vi "Begin.vi"(8 "error in":errorcluster) -> (0 "error out":errorcluster)   [LabVIEW 2016]
doc: "Called before other user functions, this VI is expected to open initial I/O refnums, load in file data, and do all program initialization. Notice that the <B>error out</B> terminal is simply used for data flow. Wiring it to other structures or subVIs ensures that this VI runs first."
uses:
  <vilib>/Rock Robotics/WPI/DriverStation/WPI_DriverStationRobotMode2.ctl
  <vilib>/Rock Robotics/WPI/Joystick/WPI_JoystickDeviceEnum.ctl
  <vilib>/Rock Robotics/WPI/ThirdParty/CanMotor/TalonSRX/WPI_CANTalonSRX_APIControlMode.ctl
  <vilib>/Rock Robotics/WPI/ThirdParty/CanMotor/TalonSRX/WPI_CANTalonSRX_BrakeOverride.ctl
  <vilib>/Rock Robotics/WPI/ThirdParty/CanMotor/TalonSRX/WPI_CANTalonSRX_APIFeedbackSelect.ctl
  <vilib>/Rock Robotics/WPI/Solenoid/WPI_SolenoidChannel.ctl
  <vilib>/Rock Robotics/WPI/Solenoid/WPI_SolenoidValue.ctl
  <vilib>/Rock Robotics/SystemInterfaces/DIO/FPGA_DIOChannel.ctl
  Robot Global Data.vi
  <vilib>/Rock Robotics/WPI/Solenoid/WPI_SolenoidOpenSingle.vi
  <vilib>/Rock Robotics/WPI/Solenoid/WPI_SolenoidSetEnum.vi
  <vilib>/Rock Robotics/WPI/Switch/WPI_SwitchOpenLimit.vi
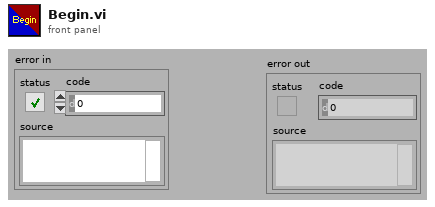
[diagram p1: front panel]
types:
  T1 = typedef "FPGA_DIOChannel.ctl" = enum8{"DIO 0", "DIO 1", "DIO 2", "DIO 3", "DIO 4", "DIO 5", "DIO 6", "DIO 7", "DIO 8", "DIO 9", "DIO MXP 0", "DIO MXP 1", "DIO MXP 2", "DIO MXP 3", "DIO MXP 4", "DIO MXP 5", "DIO MXP 6", "DIO MXP 7", "DIO MXP 8", "DIO MXP 9", "DIO MXP 10", "DIO MXP 11", "DIO MXP 12", "DIO MXP 13", "DIO MXP 14", "DIO MXP 15", "SPI Port CS1", "SPI Port CS2", "SPI Port CS3", "SPI Port MISO", "SPI Port MOSI", "Invalid"}
  T2 = typedef "WPI_SolenoidValue.ctl" = enum16{"Off", "On", "Forward", "Reverse"}
  T3 = typedef "WPI_SolenoidChannel.ctl" = enum8{"Solenoid 0", "Solenoid 1", "Solenoid 2", "Solenoid 3", "Solenoid 4", "Solenoid 5", "Solenoid 6", "Solenoid 7", "Invalid"}
  T4 = typedef "WPI_CANTalonSRX_BrakeOverride.ctl" = enum8{"No Override", "Override to Coast", "Override to Brake"}
  T5 = typedef "WPI_CANTalonSRX_APIControlMode.ctl" = enum8{"Percent VBus", "Speed", "Position", "Slave", "Unchanged / Invalid", "Voltage Compensation", "Current", "Motion Profile", "Motion Magic"}
  T6 = typedef "WPI_CANTalonSRX_APIFeedbackSelect.ctl" = enum16{"Digital Quadrature Encoder", "Analog Potentiometer", "Analog Encoder", "Count on Quad-A (Rising-Edge)", "Count on Quad-A (Falling-Edge)", "CTR Magnetic Enc (Absolute)", "CTR Magnetic Enc (Relative)", "Pulse Width"}
  T7 = typedef "WPI_JoystickDeviceEnum.ctl" = enum16{"USB 0", "USB 1", "USB 2", "USB 3", "USB 4", "USB 5"}
  T8 = typedef "WPI_DriverStationRobotMode2.ctl" = enum16{"Autonomous Disabled", "Autonomous Enabled", "Teleop Disabled", "Teleop Enabled", "Disconnected", "Finish", "Test Disabled", "Test Enabled", "Emergency Stopped"}
  T9 = typedef "WPI_JoystickDevRef.ctl" = cluster{"Device":T7}
  T10 = typedef "WPI_MotorControlDeviceRef.ctl" = cluster{"DeviceStatus":errorcluster, "Type":T11, "PWM":cluster{"PWM Channel":T12, "DeadBand":T13}, "CAN":cluster{"Device Number":u8, "SetOutput VI Ref":variant, "GetOutput VI Ref":variant, "Enable VI Ref":variant, "Disable VI Ref":variant, "Data":variant}, "Invert":bool}
  T11 = typedef "WPI_MotorControlType.ctl" = enum16{"PWM", "CAN"}
  T12 = typedef "FPGA_DIOPWMChannel.ctl" = enum8{"PWM 0", "PWM 1", "PWM 2", "PWM 3", "PWM 4", "PWM 5", "PWM 6", "PWM 7", "PWM 8", "PWM 9", "PWM MXP 0", "PWM MXP 1", "PWM MXP 2", "PWM MXP 3", "PWM MXP 4", "PWM MXP 5", "PWM MXP 6", "PWM MXP 7", "PWM MXP 8", "PWM MXP 9", "Invalid"}
  T13 = typedef "WPI_PWMDeadband.ctl" = cluster{"Name":string, "maxPositivePwm":i32, "minPositivePwm":i32, "centerPwm":i32, "maxNegativePwm":i32, "minNegativePwm":i32, "angularRange":u16}
  T14 = typedef "WPI_SwitchDevRef.ctl" = cluster{"DevStatus":errorcluster, "DIO Channel":T1, "CntIndex":T15, "Normally Closed":bool}
  T15 = typedef "FPGA_CounterCtrSystemIndex.ctl" = enum8{"Ctr 0", "Ctr 1", "Ctr 2", "Ctr 3", "Ctr 4", "Ctr 5", "Ctr 6", "Ctr 7", "Invalid"}
  T16 = typedef "WPI_SolenoidDevRef.ctl" = cluster{"DevStatus":errorcluster, "Pneumatics Control Module":u8, "Forward Solenoid Channel":T3, "Reverse Solenoid Channel":T3}
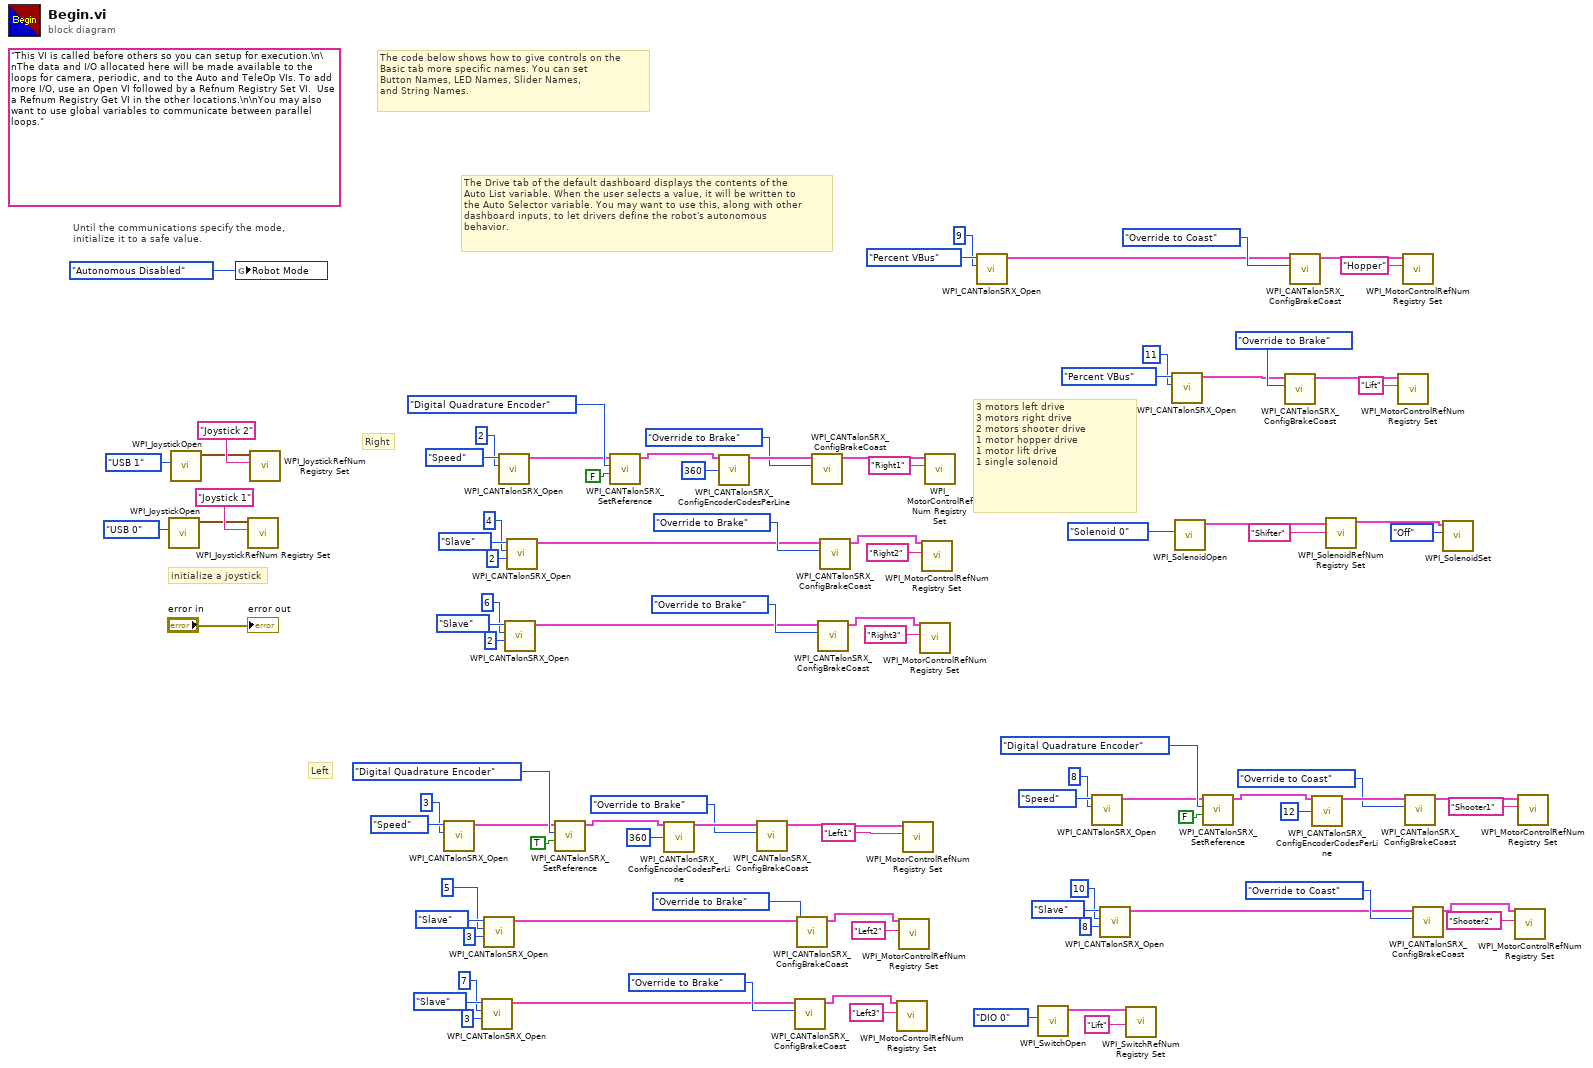
[diagram p0: block diagram]
diagram:
  (unwired) "This VI is called before others so you can setup for execution.\n\nThe data and I/O allocated here will be made available to the loops for camera, periodic, and to the Auto and TeleOp VIs. To add more I/O, use an Open VI followed by a Refnum Registry Set VI.  Use a Refnum Registry Get VI in the other locations.\n\nYou may also want to use global variables to communicate between parallel loops."
  # "3 motors left drive\n3 motors right drive\n2 motors shooter drive\n1 motor hopper drive\n1 motor lift drive\n1 single solenoid"
  # "Right"
  # "Left"
  # "The Drive tab of the default dashboard displays the contents of the\nAuto List variable. When the user selects a value, it will be written to\nthe Auto Selector variable. You may want to use this, along with other\ndashboard inputs, to let drivers define the robot's autonomous\nbehavior."
  # "The code below shows how to give controls on the\nBasic tab more specific names. You can set\nButton Names, LED Names, Slider Names,\nand String Names."
  # "initialize a joystick"
  # "Until the communications specify the mode,\ninitialize it to a safe value."
  n1 = call <vilib>:"WPI_JoystickOpen.vi"("JoystickDevice"=WPI_JoystickDeviceEnum."USB 0") -> ("JoystickDevRef"=w94:T9)  [unwired: 10 in]
  n2 = call <vilib>:"WPI_JoystickOpen.vi"("JoystickDevice"=WPI_JoystickDeviceEnum."USB 1") -> ("JoystickDevRef"=w90:T9)  [unwired: 10 in]
  n3 = global write "Robot Global Data.vi" "Robot Mode"(WPI_DriverStationRobotMode2."Autonomous Disabled" ("Robot Mode")) -> ()
  n4 = call <vilib>:"WPI_JoystickRefNum Registry Set.vi"("refnum name"="Joystick 1", "JoystickDevRef"=w94) -> ()  [unwired: 8 in, 2 out]
  n5 = call <vilib>:"WPI_JoystickRefNum Registry Set.vi"("refnum name"="Joystick 2", "JoystickDevRef"=w90) -> ()  [unwired: 8 in, 2 out]
  n6 = call <vilib>:"WPI_CANTalonSRX_Open.vi"("Device Number"=u8 3, "Control Mode"=WPI_CANTalonSRX_APIControlMode."Speed") -> ("CAN Talon SRX Ref"=w15:T10)  [unwired: 8 in, 1 out]
  n7 = call <vilib>:"WPI_CANTalonSRX_Open.vi"("Master Device Number"=u8 3, "Device Number"=u8 7, "Control Mode"=WPI_CANTalonSRX_APIControlMode."Slave") -> ("CAN Talon SRX Ref"=w66:T10)  [unwired: 7 in, 1 out]
  n8 = call <vilib>:"WPI_CANTalonSRX_Open.vi"("Master Device Number"=u8 3, "Device Number"=u8 5, "Control Mode"=WPI_CANTalonSRX_APIControlMode."Slave") -> ("CAN Talon SRX Ref"=w73:T10)  [unwired: 7 in, 1 out]
  n9 = call <vilib>:"WPI_CANTalonSRX_Open.vi"("Device Number"=u8 2, "Control Mode"=WPI_CANTalonSRX_APIControlMode."Speed") -> ("CAN Talon SRX Ref"=w81:T10)  [unwired: 8 in, 1 out]
  n10 = call <vilib>:"WPI_CANTalonSRX_Open.vi"("Master Device Number"=u8 2, "Device Number"=u8 6, "Control Mode"=WPI_CANTalonSRX_APIControlMode."Slave") -> ("CAN Talon SRX Ref"=w52:T10)  [unwired: 7 in, 1 out]
  n11 = call <vilib>:"WPI_CANTalonSRX_Open.vi"("Master Device Number"=u8 2, "Device Number"=u8 4, "Control Mode"=WPI_CANTalonSRX_APIControlMode."Slave") -> ("CAN Talon SRX Ref"=w59:T10)  [unwired: 7 in, 1 out]
  n12 = call <vilib>:"WPI_CANTalonSRX_SetReference.vi"("Reverse Feedback Sensor"=TRUE, "Feedback Reference"=WPI_CANTalonSRX_APIFeedbackSelect."Digital Quadrature Encoder", "CAN Talon SRX Ref"=w15) -> ("CAN Talon SRX Ref"=w14:T10)  [unwired: 7 in, 1 out]
  n13 = call <vilib>:"WPI_CANTalonSRX_SetReference.vi"("Reverse Feedback Sensor"=FALSE, "Feedback Reference"=WPI_CANTalonSRX_APIFeedbackSelect."Digital Quadrature Encoder", "CAN Talon SRX Ref"=w81) -> ("CAN Talon SRX Ref"=w80:T10)  [unwired: 7 in, 1 out]
  n14 = call <vilib>:"WPI_CANTalonSRX_ConfigEncoderCodesPerLine.vi"("CAN Talon SRX Ref"=w14, "Number Encoder Lines\n(Counts Per Rotation)"=u32 360 ("Number Encoder Lines\n(Counts Per Rotation)")) -> ("CAN Talon SRX Ref"=w18:T10)  [unwired: 12 in, 1 out]
  n15 = call <vilib>:"WPI_CANTalonSRX_ConfigEncoderCodesPerLine.vi"("CAN Talon SRX Ref"=w80, "Number Encoder Lines\n(Counts Per Rotation)"=u32 360 ("Number Encoder Lines\n(Counts Per Rotation)")) -> ("CAN Talon SRX Ref"=w84:T10)  [unwired: 12 in, 1 out]
  n16 = call <vilib>:"WPI_CANTalonSRX_ConfigBrakeCoast.vi"("Brake / Coast Mode"=WPI_CANTalonSRX_BrakeOverride."Override to Brake", "CAN Talon SRX Ref"=w18) -> ("CAN Talon SRX Ref"=w13:T10)  [unwired: 8 in, 1 out]
  n17 = call <vilib>:"WPI_CANTalonSRX_ConfigBrakeCoast.vi"("Brake / Coast Mode"=WPI_CANTalonSRX_BrakeOverride."Override to Brake", "CAN Talon SRX Ref"=w66) -> ("CAN Talon SRX Ref"=w67:T10)  [unwired: 8 in, 1 out]
  n18 = call <vilib>:"WPI_CANTalonSRX_ConfigBrakeCoast.vi"("Brake / Coast Mode"=WPI_CANTalonSRX_BrakeOverride."Override to Brake", "CAN Talon SRX Ref"=w73) -> ("CAN Talon SRX Ref"=w74:T10)  [unwired: 8 in, 1 out]
  n19 = call <vilib>:"WPI_CANTalonSRX_ConfigBrakeCoast.vi"("Brake / Coast Mode"=WPI_CANTalonSRX_BrakeOverride."Override to Brake", "CAN Talon SRX Ref"=w84) -> ("CAN Talon SRX Ref"=w79:T10)  [unwired: 8 in, 1 out]
  n20 = call <vilib>:"WPI_CANTalonSRX_ConfigBrakeCoast.vi"("Brake / Coast Mode"=WPI_CANTalonSRX_BrakeOverride."Override to Brake", "CAN Talon SRX Ref"=w52) -> ("CAN Talon SRX Ref"=w53:T10)  [unwired: 8 in, 1 out]
  n21 = call <vilib>:"WPI_CANTalonSRX_ConfigBrakeCoast.vi"("Brake / Coast Mode"=WPI_CANTalonSRX_BrakeOverride."Override to Brake", "CAN Talon SRX Ref"=w59) -> ("CAN Talon SRX Ref"=w60:T10)  [unwired: 8 in, 1 out]
  n22 = call <vilib>:"WPI_MotorControlRefNum Registry Set.vi"("refnum name"="Left3", "MotorControlDevRef"=w67) -> ()  [unwired: 8 in, 2 out]
  n23 = call <vilib>:"WPI_MotorControlRefNum Registry Set.vi"("refnum name"="Left2", "MotorControlDevRef"=w74) -> ()  [unwired: 8 in, 2 out]
  n24 = call <vilib>:"WPI_MotorControlRefNum Registry Set.vi"("refnum name"="Left1", "MotorControlDevRef"=w13) -> ()  [unwired: 8 in, 2 out]
  n25 = call <vilib>:"WPI_MotorControlRefNum Registry Set.vi"("refnum name"="Right3", "MotorControlDevRef"=w53) -> ()  [unwired: 8 in, 2 out]
  n26 = call <vilib>:"WPI_MotorControlRefNum Registry Set.vi"("refnum name"="Right2", "MotorControlDevRef"=w60) -> ()  [unwired: 8 in, 2 out]
  n27 = call <vilib>:"WPI_MotorControlRefNum Registry Set.vi"("refnum name"="Right1", "MotorControlDevRef"=w79) -> ()  [unwired: 8 in, 2 out]
  n28 = call <vilib>:"WPI_CANTalonSRX_Open.vi"("Device Number"=u8 9, "Control Mode"=WPI_CANTalonSRX_APIControlMode."Percent VBus") -> ("CAN Talon SRX Ref"=w10:T10)  [unwired: 8 in, 1 out]
  n29 = call-poly <vilib>:"WPI_SwitchOpen.vi"("DIO Channel"=FPGA_DIOChannel."DIO 0") -> ("SwitchDevRef"=w2:T14)  [unwired: 9 in, 1 out]
  n30 = call <vilib>:"WPI_CANTalonSRX_Open.vi"("Device Number"=u8 8, "Control Mode"=WPI_CANTalonSRX_APIControlMode."Speed") -> ("CAN Talon SRX Ref"=w43:T10)  [unwired: 8 in, 1 out]
  n31 = call <vilib>:"WPI_CANTalonSRX_Open.vi"("Master Device Number"=u8 8, "Device Number"=u8 10, "Control Mode"=WPI_CANTalonSRX_APIControlMode."Slave") -> ("CAN Talon SRX Ref"=w34:T10)  [unwired: 7 in, 1 out]
  n32 = call <vilib>:"WPI_SwitchRefNum Registry Set.vi"("refnum name"="Lift", "SwitchDevRef"=w2) -> ()  [unwired: 8 in, 2 out]
  n33 = call <vilib>:"WPI_CANTalonSRX_Open.vi"("Device Number"=u8 11, "Control Mode"=WPI_CANTalonSRX_APIControlMode."Percent VBus") -> ("CAN Talon SRX Ref"=w9:T10)  [unwired: 8 in, 1 out]
  n34 = call-poly <vilib>:"WPI_SolenoidOpen.vi"("Solenoid Channel"=WPI_SolenoidChannel."Solenoid 0") -> ("SolenoidDevRef"=w7:T16)  [unwired: 9 in, 1 out]
  n35 = call <vilib>:"WPI_CANTalonSRX_SetReference.vi"("Reverse Feedback Sensor"=FALSE, "Feedback Reference"=WPI_CANTalonSRX_APIFeedbackSelect."Digital Quadrature Encoder", "CAN Talon SRX Ref"=w43) -> ("CAN Talon SRX Ref"=w42:T10)  [unwired: 7 in, 1 out]
  n36 = call <vilib>:"WPI_CANTalonSRX_ConfigBrakeCoast.vi"("Brake / Coast Mode"=WPI_CANTalonSRX_BrakeOverride."Override to Brake", "CAN Talon SRX Ref"=w9) -> ("CAN Talon SRX Ref"=w24:T10)  [unwired: 8 in, 1 out]
  n37 = call <vilib>:"WPI_CANTalonSRX_ConfigBrakeCoast.vi"("Brake / Coast Mode"=WPI_CANTalonSRX_BrakeOverride."Override to Coast", "CAN Talon SRX Ref"=w10) -> ("CAN Talon SRX Ref"=w29:T10)  [unwired: 8 in, 1 out]
  n38 = call <vilib>:"WPI_CANTalonSRX_ConfigEncoderCodesPerLine.vi"("CAN Talon SRX Ref"=w42, "Number Encoder Lines\n(Counts Per Rotation)"=u32 12 ("Number Encoder Lines\n(Counts Per Rotation)")) -> ("CAN Talon SRX Ref"=w46:T10)  [unwired: 12 in, 1 out]
  n39 = call <vilib>:"WPI_SolenoidRefNum Registry Set.vi"("refnum name"="Shifter", "SolenoidDevRef"=w7) -> ("SolenoidDevRef"=w6:T16)  [unwired: 8 in, 1 out]
  n40 = call <vilib>:"WPI_MotorControlRefNum Registry Set.vi"("refnum name"="Lift", "MotorControlDevRef"=w24) -> ()  [unwired: 8 in, 2 out]
  n41 = call <vilib>:"WPI_MotorControlRefNum Registry Set.vi"("refnum name"="Hopper", "MotorControlDevRef"=w29) -> ()  [unwired: 8 in, 2 out]
  n42 = call <vilib>:"WPI_CANTalonSRX_ConfigBrakeCoast.vi"("Brake / Coast Mode"=WPI_CANTalonSRX_BrakeOverride."Override to Coast", "CAN Talon SRX Ref"=w46) -> ("CAN Talon SRX Ref"=w41:T10)  [unwired: 8 in, 1 out]
  n43 = call <vilib>:"WPI_CANTalonSRX_ConfigBrakeCoast.vi"("Brake / Coast Mode"=WPI_CANTalonSRX_BrakeOverride."Override to Coast", "CAN Talon SRX Ref"=w34) -> ("CAN Talon SRX Ref"=w35:T10)  [unwired: 8 in, 1 out]
  n44 = call-poly <vilib>:"WPI_SolenoidSet.vi"("Value"=WPI_SolenoidValue."Off", "SolenoidDevRef"=w6) -> ()  [unwired: 8 in, 2 out]
  n45 = call <vilib>:"WPI_MotorControlRefNum Registry Set.vi"("refnum name"="Shooter2", "MotorControlDevRef"=w35) -> ()  [unwired: 8 in, 2 out]
  n46 = call <vilib>:"WPI_MotorControlRefNum Registry Set.vi"("refnum name"="Shooter1", "MotorControlDevRef"=w41) -> ()  [unwired: 8 in, 2 out]
  "error out" <- "error in"
